vi "Parameters_GetPositionParams.vi"(11 "Parameters":dbl[](array[numeric])) -> (0 "Acceleration Jerk":dbl=1000.0, 1 "Acceleration":dbl=10000.0, 2 "Velocity":dbl=1000.0, 3 "Target Position":dbl)   [LabVIEW 2017, in "WordManipulationLibrary.lvlib"]
uses:
  WordManipulationLibrary.lvlib
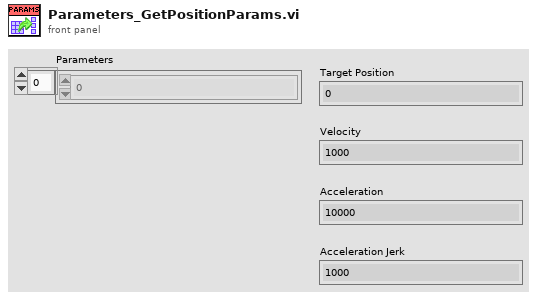
[diagram p1: front panel]
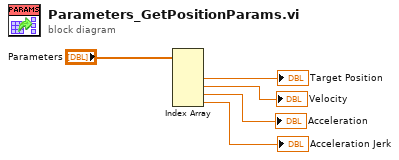
[diagram p0: block diagram]
diagram:
  n1 = Index Array(array="Parameters") -> (element #2=→"Target Position":dbl, element #3=→"Velocity":dbl, element #4=→"Acceleration":dbl, element #5=→"Acceleration Jerk":dbl)  [unwired: 5 in, 1 out]
